vi "Configure Modulation Table.vi"(0 "VISA resource name":refnum<visa-resource-name>, 1 "VMOD":dbl min=0.0 max=9999.0 step=0.001, 2 "Mod":dbl min=-1000.0 max=1000.0 step=0.001, 5 "Modulation":u32(ring) items=["Not Available", "Available"], 9 "Row":u32=1 min=1 max=50 step=1, 11 "error in (no error)":errorcluster, 12 "Loc":u32 max=1 step=1) -> (4 "VISA resource name out":refnum<visa-resource-name>, 15 "error out":errorcluster)   [LabVIEW 2022 SP3, in "MagnaDC.lvlib"]
uses:
  MagnaDC.lvlib
panel:
  # "Modulation Table Row"
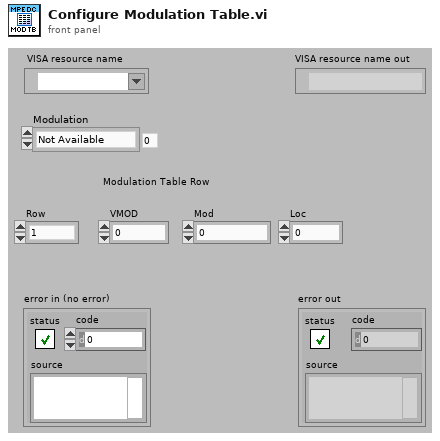
[diagram p1: front panel]
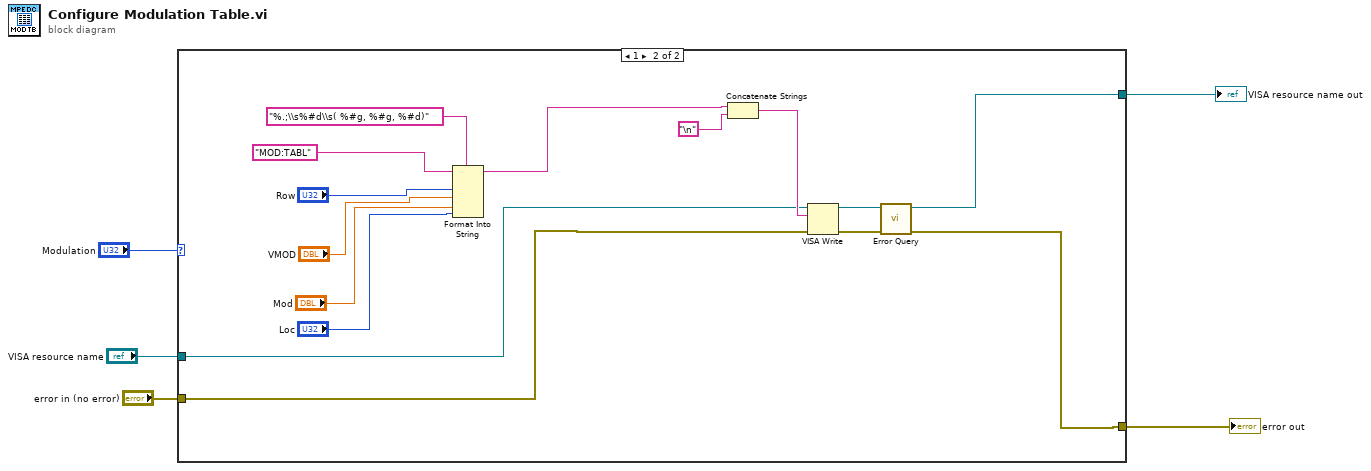
[diagram p0: block diagram]
diagram:
  n1 = case shown="1" "Modulation" {
    tunnel: "VISA resource name" -> [w6 w9]
    tunnel: "error in (no error)" -> [w7 w8]
    tunnel: [w6 w11] -> w2
    tunnel: [w7 w10] -> w1
    frame 0, Default {
    }
    frame 1 {
      n2 = Format Into String(format string="%.;\\s%#d\\s( %#g, %#g, %#d)", initial string="MOD:TABL", "Row", "VMOD", "Mod", "Loc") -> (resulting string=w12:string)  [unwired: 1 in, 1 out]
      n3 = Concatenate Strings(w12, "\n") -> (w13:string)
      n4 = VISA Write(VISA resource name=w9, write buffer=w13, error in (no error)=w8) -> (VISA resource name out=w16:refnum<visa-resource-name>, error out=w15:errorcluster)  [unwired: 1 out]
      n5 = call "Error Query.vi"("error in (no error)"=w15, "VISA resource name"=w16) -> ("error out"=w10:errorcluster, "VISA resource name out"=w11:refnum<visa-resource-name>)  [unwired: 6 in, 2 out]
    }
  }
  "error out" <- w1
  "VISA resource name out" <- w2
